vi "trapControl.vi"() -> ()   [LabVIEW 2012]
uses:
  <vilib>/DAQmx/read.llb/DAQmx Read (Counter U32 1Chan 1Samp).vi
  <vilib>/DAQmx/miscellaneous.llb/DAQmx Fill In Error Info.vi
panel:
  in  "UV Firing delay":i32=2000
  out "mean":i32
  in  "Rescale Window?":bool
  in  "X window size":dbl=5.0
  in  "Pockel":bool=TRUE
  in  "Dump Frequency":dbl
  in  "AutoDump":bool
  in  "UV":bool
  in  "1762":bool
  in  "455 LED":bool
  in  "399 Yb Ionizer":bool
  in  "Oven":bool
  in  "Orange":bool=TRUE
  in  "Sample Time":dbl=0.02 format="%0.2f"
  in  "RF":bool
  in  "Blue":bool=TRUE
  in  "Red":bool=TRUE
  in  "Samples per averaging\nblock":i32=20 min=1 step=1
  in  "stop":bool
  out "PMT Counts":cluster{"mean":dbl, u32}(graph)
  # "Macro Trap"
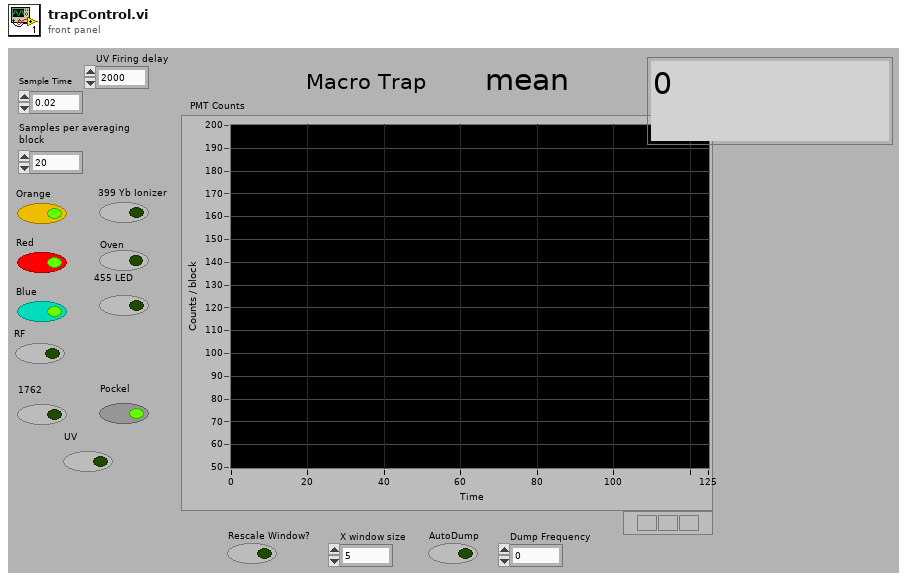
[diagram p1: front panel]
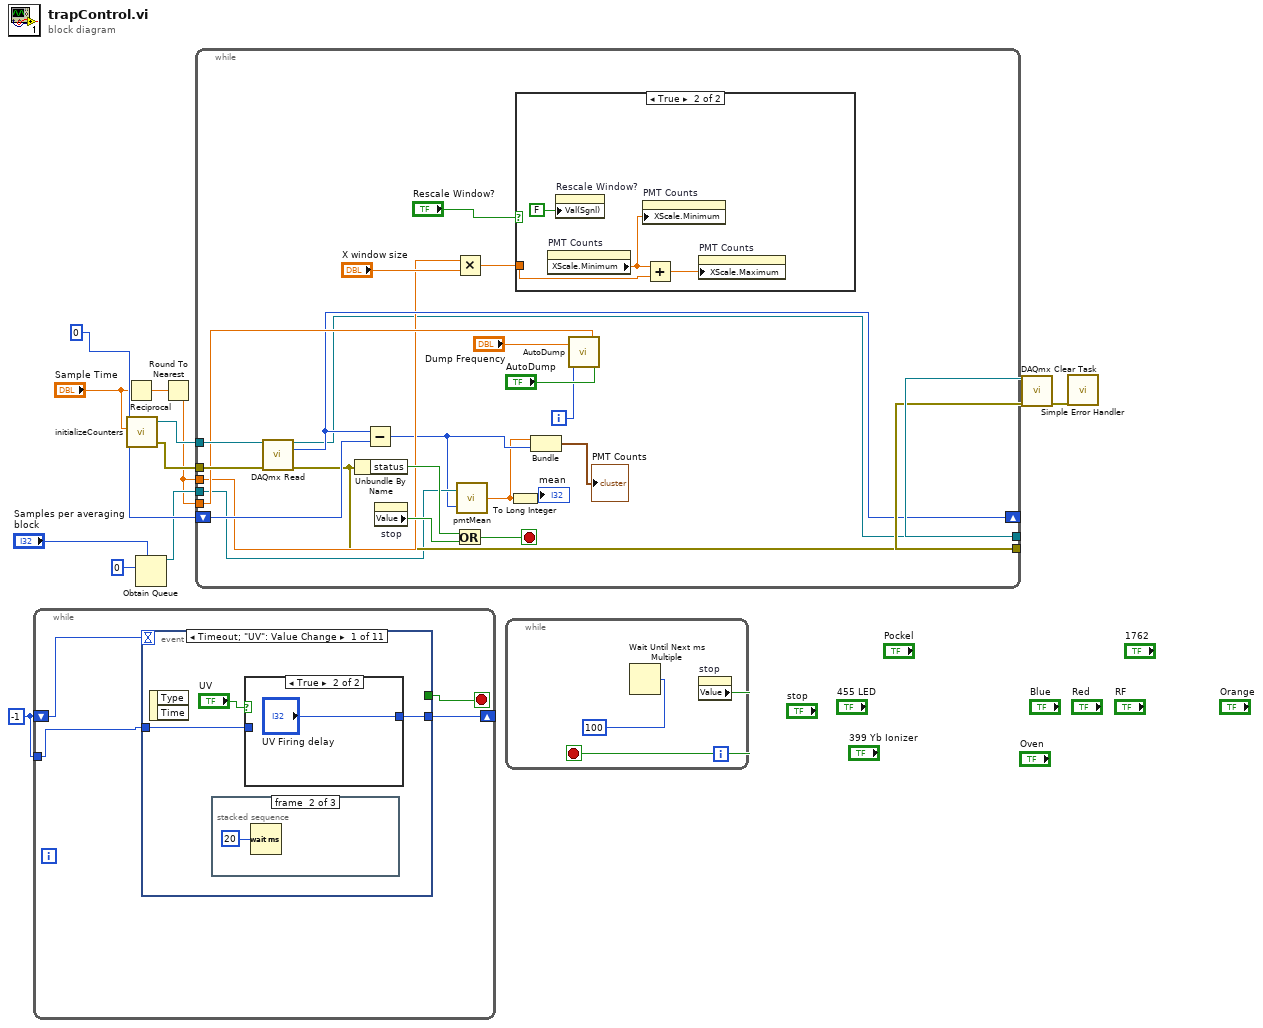
[diagram p0: block diagram]
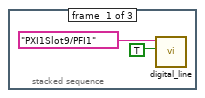
[diagram p2: hidden frame]
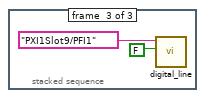
[diagram p3: hidden frame]
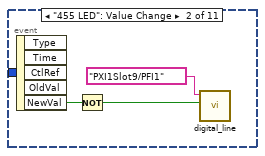
[diagram p5: hidden frame]
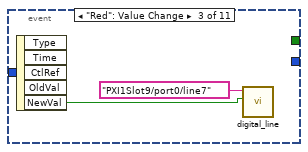
[diagram p6: hidden frame]
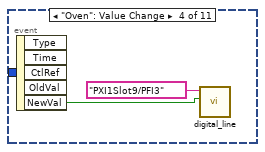
[diagram p7: hidden frame]
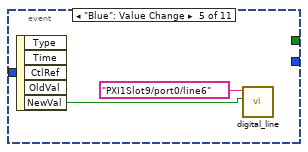
[diagram p8: hidden frame]
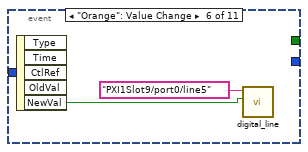
[diagram p9: hidden frame]
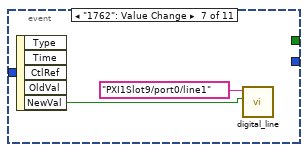
[diagram p10: hidden frame]
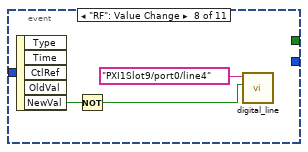
[diagram p11: hidden frame]
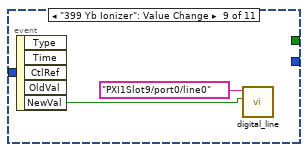
[diagram p12: hidden frame]
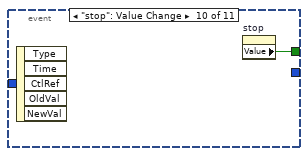
[diagram p13: hidden frame]
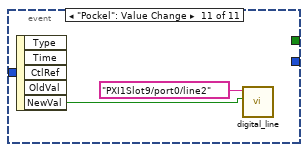
[diagram p14: hidden frame]
diagram:
  w1 = -1
  n1 = while {
    shift-right: [w16] -> _
    shift-left: w1 -> [w15]
    tunnel: w1 -> [w14]
    stop <- w17 stop-if-true
    n2 = event shown="[0] Timeout;  \"UV\": Value Change" {
      selector: _ -> [_ _ _ _ _ _ _ _ _ _ _]
      dyn-events: _ -> [_ _ _ _ _ _ _ _ _ _ _]
      timeout: w15 -> [_ _ _ _ _ _ _ _ _ _ _]
      tunnel: [_ _ _ _ _ _ _ _ _ w46 _] -> w17
      tunnel: [w20 _ _ _ _ _ _ _ _ _ _] -> w16
      tunnel: w14 -> [w19 _ _ _ _ _ _ _ _ _ _]
      event Timeout; "UV": Value Change {
        n3 = event-data() -> ()  [unwired: 1 in, 2 out]
        n4 = stacked-sequence {
          frame #0 {
            n5 = call "digital_line.vi"("Boolean"=TRUE, "lines"=tag "PXI1Slot9/PFI1") -> ()  [unwired: 5 in, 1 out]
          }
          frame #1 {
            n6 = Wait (ms)(milliseconds to wait=u32 20) -> ()  [unwired: 1 out]
          }
          frame #2 {
            n7 = call "digital_line.vi"("Boolean"=FALSE, "lines"=tag "PXI1Slot9/PFI1") -> ()  [unwired: 5 in, 1 out]
          }
        }
        n8 = case shown="True" "UV" {
          tunnel: [w26 "UV Firing delay"] -> w20
          tunnel: w19 -> [w26 _]
          frame False {
          }
          frame True {
          }
        }
      }
      event "455 LED": Value Change {
        n9 = event-data() -> ("NewVal"=w30:bool)  [unwired: 1 in, 4 out]
        n10 = Not(x=w30) -> (.not. x?=w28:bool)
        n11 = call "digital_line.vi"("Boolean"=w28, "lines"=tag "PXI1Slot9/PFI1") -> ()  [unwired: 5 in, 1 out]
      }
      event "Red": Value Change {
        n12 = event-data() -> ("NewVal"=w31:bool)  [unwired: 1 in, 4 out]
        n13 = call "digital_line.vi"("Boolean"=w31, "lines"=tag "PXI1Slot9/port0/line7") -> ()  [unwired: 5 in, 1 out]
      }
      event "Oven": Value Change {
        n14 = event-data() -> ("NewVal"=w33:bool)  [unwired: 1 in, 4 out]
        n15 = call "digital_line.vi"("Boolean"=w33, "lines"=tag "PXI1Slot9/PFI3") -> ()  [unwired: 5 in, 1 out]
      }
      event "Blue": Value Change {
        n16 = event-data() -> ("NewVal"=w35:bool)  [unwired: 1 in, 4 out]
        n17 = call "digital_line.vi"("Boolean"=w35, "lines"=tag "PXI1Slot9/port0/line6") -> ()  [unwired: 5 in, 1 out]
      }
      event "Orange": Value Change {
        n18 = event-data() -> ("NewVal"=w37:bool)  [unwired: 1 in, 4 out]
        n19 = call "digital_line.vi"("Boolean"=w37, "lines"=tag "PXI1Slot9/port0/line5") -> ()  [unwired: 5 in, 1 out]
      }
      event "1762": Value Change {
        n20 = event-data() -> ("NewVal"=w39:bool)  [unwired: 1 in, 4 out]
        n21 = call "digital_line.vi"("Boolean"=w39, "lines"=tag "PXI1Slot9/port0/line1") -> ()  [unwired: 5 in, 1 out]
      }
      event "RF": Value Change {
        n22 = event-data() -> ("NewVal"=w43:bool)  [unwired: 1 in, 4 out]
        n23 = Not(x=w43) -> (.not. x?=w41:bool)
        n24 = call "digital_line.vi"("Boolean"=w41, "lines"=tag "PXI1Slot9/port0/line4") -> ()  [unwired: 5 in, 1 out]
      }
      event "399 Yb Ionizer": Value Change {
        n25 = event-data() -> ("NewVal"=w44:bool)  [unwired: 1 in, 4 out]
        n26 = call "digital_line.vi"("Boolean"=w44, "lines"=tag "PXI1Slot9/port0/line0") -> ()  [unwired: 5 in, 1 out]
      }
      event "stop": Value Change {
        n27 = event-data() -> ()  [unwired: 1 in, 5 out]
        n28 = property on="stop" class="Bool (strict)"() -> ("Value"=w46:bool)  [unwired: 2 in, 2 out]
      }
      event "Pockel": Value Change {
        n29 = event-data() -> ("NewVal"=w47:bool)  [unwired: 1 in, 4 out]
        n30 = call "digital_line.vi"("Boolean"=w47, "lines"=tag "PXI1Slot9/port0/line2") -> ()  [unwired: 5 in, 1 out]
      }
    }
  }
  n31 = Reciprocal(x="Sample Time") -> (1/x=w8:dbl)
  n32 = call "initializeCounters.vi"("Sample Time"="Sample Time") -> ("error out"=w5:errorcluster, "task out"=w6:refnum<k21>)  [unwired: 4 in]
  n33 = Obtain Queue(max queue size (-1, unlimited)="Samples per averaging\nblock", element data type=u32 0) -> (queue out=w10:refnum<queue>)  [unwired: 3 in, 2 out]
  n34 = Round To Nearest(number=w8) -> (nearest integer value=w4:dbl)
  n35 = while {
    shift-right: [w58] -> _
    shift-left: u32 0 -> [w66]
    tunnel: w6 -> [w68]
    tunnel: w10 -> [w53]
    tunnel: w5 -> [w65]
    tunnel: w4 -> [w60]
    tunnel: w4 -> [w57]
    tunnel: [w55] -> w3
    tunnel: [w54] -> w2
    i -> [w49]
    stop <- w70 stop-if-true
    n36 = call-poly <vilib>:"DAQmx Read.vi"("task/channels in"=w68, "error in"=w65) -> ("task out"=w55:refnum<k21>, "data"=w58:u32, "error out"=w54:errorcluster)  [unwired: 11 in]
    n37 = Unbundle By Name(w54) -> ("status"=w69:bool)
    n38 = Subtract(x=w58, y=w66) -> (x-y=w52:u32)
    n39 = property on="stop" class="Bool (strict)"() -> ("Value"=w67:bool)  [unwired: 2 in, 2 out]
    n40 = Multiply(x=w57, y="X window size") -> (x*y=w63:dbl)
    n41 = Or(x=w69, y=w67) -> (x .or. y?=w70:bool)
    n42 = call "pmtMean.vi"("pmt counts"=w52, "input queue"=w53) -> ("mean"=w51:dbl)
    n43 = To Long Integer(number=w51) -> (32bit integer=→"mean":i32)
    n44 = case shown="True" "Rescale Window?" {
      tunnel: w63 -> [_ w72]
      frame False {
      }
      frame True {
        n45 = property on="PMT Counts" class="WFChart (strict)"() -> ("XScale.Minimum"=w74:dbl)  [unwired: 2 in, 2 out]
        n46 = property on="Rescale Window?" class="Bool (strict)"("Val(Sgnl)"=FALSE ("Value (Signaling)")) -> ()  [unwired: 2 in, 2 out]
        n47 = property on="PMT Counts" class="WFChart (strict)"("XScale.Minimum"=w74) -> ()  [unwired: 2 in, 2 out]
        n48 = Add(x=w74, y=w72) -> (x+y=w73:dbl)
        n49 = property on="PMT Counts" class="WFChart (strict)"("XScale.Maximum"=w73) -> ()  [unwired: 2 in, 2 out]
      }
    }
    n50 = Bundle("mean"=w51, w52) -> (→"PMT Counts":cluster{"mean":dbl, u32})  [unwired: 1 in]
    n51 = call "AutoDump.vi"("Sample Rate"=w60, "Dump Frequency"="Dump Frequency", "AutoDump"="AutoDump", "loopIteration"=w49) -> ()  [unwired: 1 in]
  }
  n52 = while {
    stop <- w75 stop-if-true
    n53 = Wait Until Next ms Multiple(millisecond multiple=u32 100) -> ()  [unwired: 1 out]
    n54 = property on="stop" class="Bool (strict)"() -> ("Value"=w75:bool)  [unwired: 2 in, 2 out]
  }
  n55 = call <vilib>:"DAQmx Clear Task.vi"("task in"=w3, "error in"=w2) -> ("error out"=w9:errorcluster)  [unwired: 13 in]
  n56 = call <vilib>:"Simple Error Handler.vi"("error in (no error)"=w9) -> ()  [unwired: 4 in, 5 out]
